vi "Dpc Clear Config Status.vi"(8 "error in (no error)":errorcluster, 9 "perc":i32, 10 "trid":u16, 11 "hif":u32) -> (0 "error out":errorcluster, 1 "perc out":i32, 2 "function return":i32, 3 "hif out":u32)   [LabVIEW 2011, in "LVH-Adept.lvlib" / "DPCUTIL.lvlib"]
doc: "DPCAPI BOOL DpcClearConfigStatus(HANDLE hif, TRID trid, ERC * perc);"
uses:
  DPCUTIL.lvlib
  Resources/dpcutil.dll
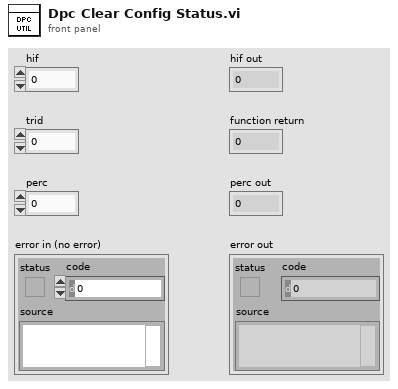
[diagram p1: front panel]
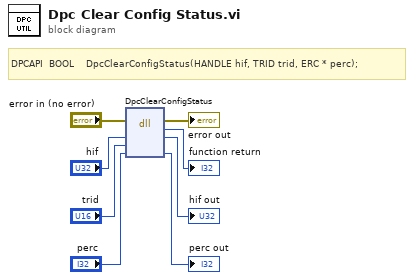
[diagram p0: block diagram]
diagram:
  # "DPCAPI  BOOL    DpcClearConfigStatus(HANDLE hif, TRID trid, ERC * perc);"
  n1 = dll-call lib="C:/github/labviewhacker/LVH-Adept/LabVIEW/vi.lib/LabVIEW Hacker/Adept/Private/Resources/dpcutil.*" fn="DpcClearConfigStatus"(error in="error in (no error)", "hif"="hif", "trid"="trid", "perc"="perc") -> (error out=→"error out":errorcluster, →"function return":i32, "hif"=→"hif out":u32, "perc"=→"perc out":i32)  [unwired: 3 in, 1 out]
